vi "Logos.vi"(8 "Fehler (Eingang, kein Fehler)":errorcluster) -> (0 "Fehler (Ausgang)":errorcluster, 1 "Default  Header Image File Path":path, 2 "Footer Image File Path":path, 3 "Header Image File Path":path)   [LabVIEW 2020, in "PDF Interface.lvlib"]
uses:
  PDF Interface.lvlib
  Allgemein/allgemeine Sub-VIs.lvlib
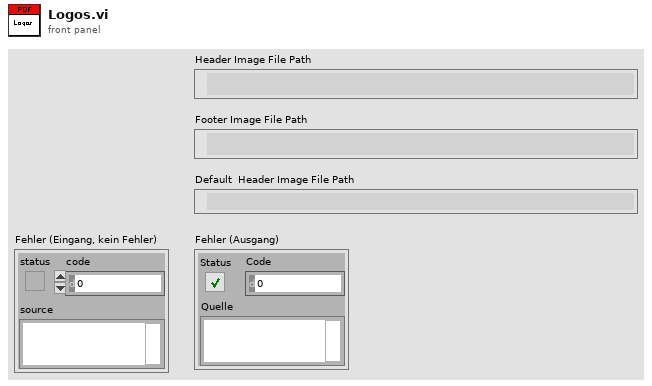
[diagram p1: front panel]
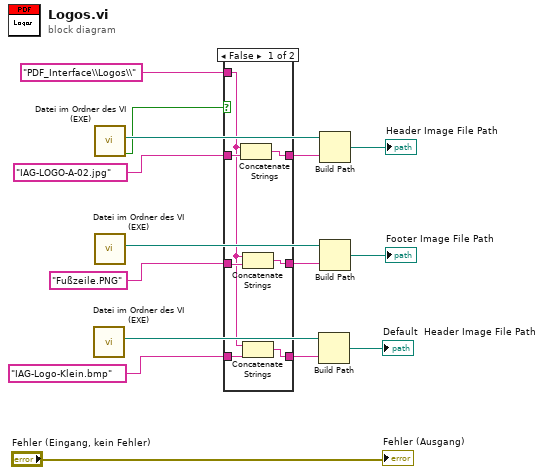
[diagram p0: block diagram]
diagram:
  n1 = call "Datei im Ordner des VI (EXE).vi"() -> ("Ordner des Haupt-VIs"=w11:path)  [unwired: 9 in, 2 out]
  n2 = call "Datei im Ordner des VI (EXE).vi"() -> ("EXE"=w9:bool, "Ordner des Haupt-VIs"=w15:path)  [unwired: 9 in, 1 out]
  n3 = call "Datei im Ordner des VI (EXE).vi"() -> ("Ordner des Haupt-VIs"=w14:path)  [unwired: 9 in, 2 out]
  n4 = case shown="False" w9 {
    tunnel: [w22 w25] -> w8
    tunnel: "IAG-LOGO-A-02.jpg" ("name or relative path") -> [w21 w25]
    tunnel: "Fußzeile.PNG" ("name or relative path") -> [w20 w24]
    tunnel: [w19 w24] -> w5
    tunnel: "IAG-Logo-Klein.bmp" ("name or relative path") -> [w18 w23]
    tunnel: [w16 w23] -> w3
    tunnel: "PDF_Interface\\Logos\\" -> [w17 _]
    frame False {
      n5 = Concatenate Strings(w17, w21) -> (w22:string)
      n6 = Concatenate Strings(w17, w20) -> (w19:string)
      n7 = Concatenate Strings(w17, w18) -> (w16:string)
    }
    frame True {
    }
  }
  n8 = Build Path(base path=w11, name or relative path=w3) -> (appended path=→"Default  Header Image File Path":path)
  n9 = Build Path(base path=w15, name or relative path=w8) -> (appended path=→"Header Image File Path":path)
  n10 = Build Path(base path=w14, name or relative path=w5) -> (appended path=→"Footer Image File Path":path)
  "Fehler (Ausgang)" <- "Fehler (Eingang, kein Fehler)"
